vi "square bracket regex.vi"(11 "string in":string) -> (1 "일치 구문 뒤":string, 2 "전체 일치 구문":string, 3 "일치 구문 앞":string)   [LabVIEW 2018, in "Library-DataConvert.lvlib"]
uses:
  Library-DataConvert.lvlib
  <vilib>/regexp/Match Regular Expression.xnode
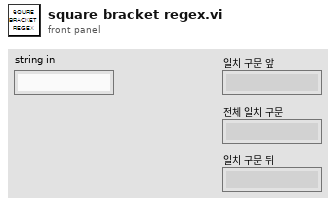
[diagram p1: front panel]
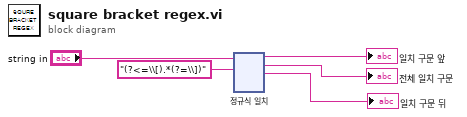
[diagram p0: block diagram]
diagram:
  n1 = xnode "정규식 일치"("입력 문자열"="string in", "정규식"="(?<=\\[).*(?=\\])") -> ("일치 구문 앞"=→"일치 구문 앞":string, "전체 일치 구문"=→"전체 일치 구문":string, "일치 구문 뒤"=→"일치 구문 뒤":string)  [unwired: 4 in, 2 out]
